vi "MakeNewFileName.vi"(8 "ErrorIn":errorcluster, 10 "Dir":path, 11 "SeriesString":string) -> (0 "ErrorOut":errorcluster, 3 "NewFileName":string)   [LabVIEW 2019]
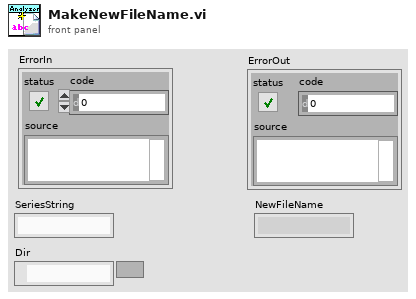
[diagram p1: front panel]
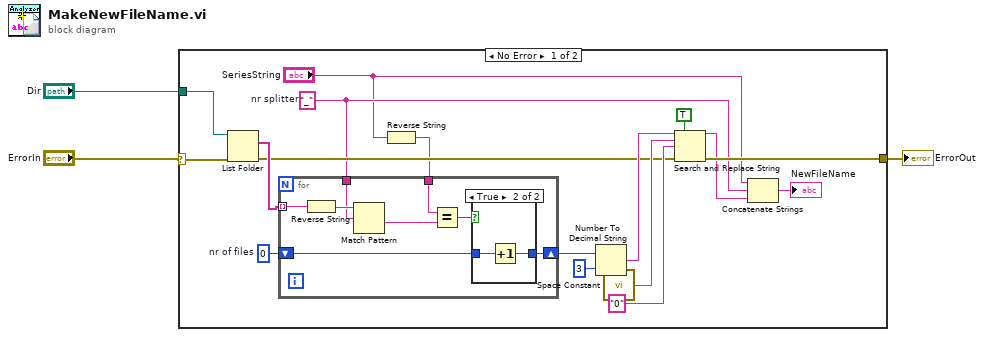
[diagram p0: block diagram]
diagram:
  n1 = case shown="No Error" "ErrorIn" {
    selector: "ErrorIn" -> [w4 w32]
    tunnel: "Dir" -> [w20 _]
    tunnel: [w10 w32] -> w2
    frame No Error {
      w18 = 0  # nr of files
      w8 = "_"  # nr splitter
      n2 = List Folder(path=w20, error in=w4) -> (filenames=w19:string[], error out=w11:errorcluster)  [unwired: 2 in, 2 out]
      n3 = Reverse String(1:"SeriesString") -> (0:w6:string)
      n4 = for {
        tunnel: w19 -> [w28] mode=indexing
        tunnel: w8 -> [w26]
        tunnel: w6 -> [w24]
        shift-right: [w21] -> w12
        shift-left: w18 -> [w22]
        n5 = Reverse String(1:w28) -> (0:w27:string)
        n6 = Match Pattern(string=w27, regular expression=w26) -> (after substring=w25:string)  [unwired: 1 in, 3 out]
        n7 = Equal?(x=w24, y=w25) -> (x = y?=w23:bool)
        n8 = case shown="True" w23 {
          tunnel: w22 -> [w29 w31]
          tunnel: [w29 w30] -> w21
          frame False {
          }
          frame True {
            n9 = Increment(x=w31) -> (x+1=w30:i32)
          }
        }
      }
      n10 = Number To Decimal String(number=w12, width (-)=i16 3) -> (decimal integer string=w16:string)
      n11 = call <vilib>:"Space Constant.vi"() -> ("String"=w14:string)
      n12 = Search and Replace String(replace all?=TRUE ("replace all? (F)"), input string=w16, search string=w14, replace string="0" ("replace string (\"\")"), error in=w11) -> (result string=w9:string, error out=w10:errorcluster)  [unwired: 3 in, 2 out]
      n13 = Concatenate Strings("SeriesString", w8, w9) -> (→"NewFileName":string)
    }
    frame Error {
    }
  }
  "ErrorOut" <- w2
